vi "Filter Check.vi"(10 "Cross CSM Data in":T1, 11 "GlobalLogFilter in":refnum<class "GlobalLogFilter.lvclass">) -> (0 "Matched? (dup)":bool, 2 "Cross CSM Data out":T1, 3 "GlobalLogFilter.lvclass (dup)":refnum<class "GlobalLogFilter.lvclass">)   [LabVIEW 2017]
uses:
  _Support/Typedef/_CSM_GlobalLog_MSG.ctl
  _Support/Typedef/_CSM_Response Source Message.ctl
  _Support/Typedef/_CSM_GlobalLog_MSG_TYPE.ctl
  GlobalLogFilter.lvclass
  Communicable State Machine.lvlib
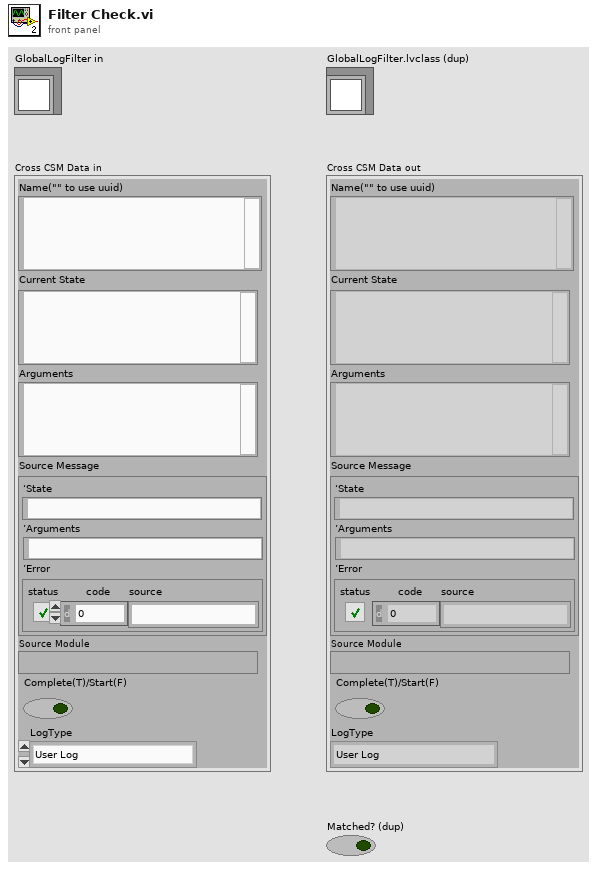
[diagram p1: front panel]
types:
  T1 = typedef "Communicable State Machine.lvlib/_CSM_GlobalLog_MSG.ctl" = cluster{"Name(\"\" to use uuid)":string, "Current State":string, "Arguments":string, "Source Message":T2, "Source Module":string, "Complete(T)/Start(F)":bool, "LogType":T3}
  T2 = typedef "Communicable State Machine.lvlib/_CSM_Response Source Message.ctl" = cluster{"‘State":string, "’Arguments":string, "’Error":errorcluster}
  T3 = typedef "Communicable State Machine.lvlib/_CSM_GlobalLog_MSG_TYPE.ctl" = enum16{"User Log", "State Change", "Status", "Interrupt", "Register", "Unregister", "Error Log", "Module Created", "Module Destroyed"}
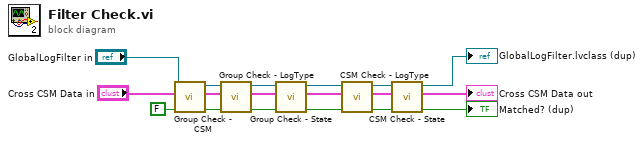
[diagram p0: block diagram]
diagram:
  n1 = call "Group Check - CSM.vi"("Matched Previous?"=FALSE, "Cross CSM Data (in)"="Cross CSM Data in", "GlobalLogFilter.lvclass"="GlobalLogFilter in") -> ("Matched? (dup)"=w12:bool, "Cross CSM Data"=w11:T1, "GlobalLogFilter.lvclass (dup)"=w10:refnum<class "GlobalLogFilter.lvclass">)  [unwired: 6 in]
  n2 = call "Group Check - LogType.vi"("Matched Previous?"=w12, "Cross CSM Data (in)"=w11, "GlobalLogFilter.lvclass"=w10) -> ("Matched? (dup)"=w18:bool, "Cross CSM Data"=w14:T1, "GlobalLogFilter.lvclass (dup)"=w17:refnum<class "GlobalLogFilter.lvclass">)  [unwired: 6 in]
  n3 = call "Group Check - State.vi"("Matched Previous?"=w18, "Cross CSM Data (in)"=w14, "GlobalLogFilter.lvclass"=w17) -> ("Matched? (dup)"=w6:bool, "Cross CSM Data"=w9:T1, "GlobalLogFilter.lvclass (dup)"=w3:refnum<class "GlobalLogFilter.lvclass">)  [unwired: 6 in]
  n4 = call "CSM Check - LogType.vi"("Matched Previous?"=w6, "Cross CSM Data (in)"=w9, "GlobalLogFilter.lvclass"=w3) -> ("Matched? (dup)"=w5:bool, "Cross CSM Data"=w8:T1, "GlobalLogFilter.lvclass (dup)"=w7:refnum<class "GlobalLogFilter.lvclass">)  [unwired: 6 in]
  n5 = call "CSM Check - State.vi"("Matched Previous?"=w5, "Cross CSM Data (in)"=w8, "GlobalLogFilter.lvclass"=w7) -> ("Matched? (dup)"=→"Matched? (dup)":bool, "Cross CSM Data"=→"Cross CSM Data out":T1, "GlobalLogFilter.lvclass (dup)"=→"GlobalLogFilter.lvclass (dup)":refnum<class "GlobalLogFilter.lvclass">)  [unwired: 6 in]
